vi "auto_detect_arduino.vi"(0 "instr name":string="Arduino Micro" caption="Arduino Board Name", 1 "error in":errorcluster) -> (2 "VISA resource name":refnum<visa-resource-name>, 3 "status":bool, 4 "error out":errorcluster)   [LabVIEW 2013]
uses:
  <vilib>/Instr/_visa.llb/VISA Find Search Mode.ctl
  <vilib>/regexp/Match Regular Expression.xnode
panel:
  # "Auto Detect ARDUINO"
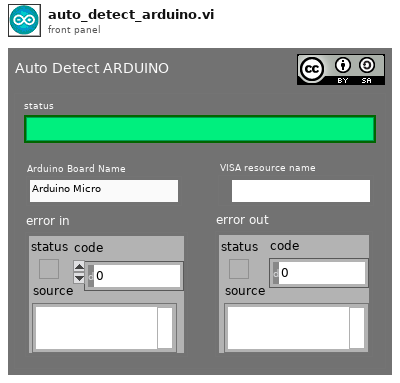
[diagram p1: front panel]
types:
  T1 = typedef "VISA Find Search Mode.ctl" = u32
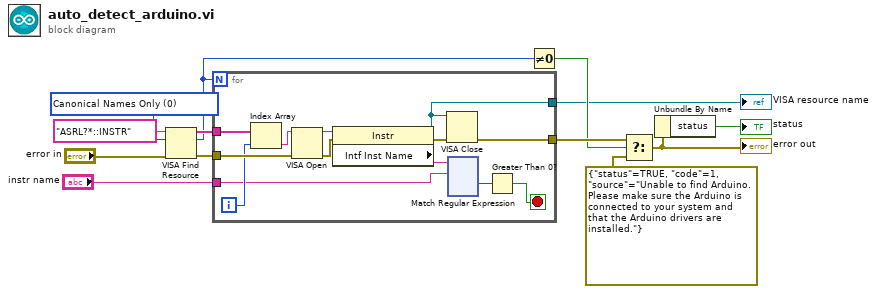
[diagram p0: block diagram]
diagram:
  w1 = T1 0 items=["Canonical Names Only"=0, "Aliases Only"=2, "Include Matching Aliases"=3, "Include All Aliases"=4] ("Search Mode")
  n1 = VISA Find Resource(8:"error in", 10:w1, 11:"ASRL?*::INSTR" ("expression (\"?*\")")) -> (0:w3:errorcluster, 2:w2:u32, 3:w4:string[])
  n2 = for {
    N: w2 -> [_]
    tunnel: w4 -> [w26]
    tunnel: w3 -> [w25]
    tunnel: [w17] -> w7
    tunnel: [w24] -> w13
    tunnel: "instr name" -> [w14]
    i -> [w23]
    stop <- w15 stop-if-true
    n3 = Index Array(array=w26, index=w23) -> (element=w22:string)
    n4 = VISA Open(error in (no error)=w25, VISA resource name=w22) -> (VISA resource name=w21:refnum<visa-resource-name>, error out=w20:errorcluster)  [unwired: 3 in]
    n5 = property class="Instr"(reference=w21, error in=w20) -> (reference out=w17:refnum<visa-resource-name>, error out=w19:errorcluster, "Intf Inst Name"=w16:string)
    n6 = VISA Close(VISA resource name=w17, error in (no error)=w19) -> (error out=w24:errorcluster)
    n7 = xnode "Match Regular Expression"("input string"=w16, "regular expression"=w14) -> ("offset past match"=w18:i32)  [unwired: 4 in, 4 out]
    n8 = Greater Than 0?(x=w18) -> (x > 0?=w15:bool)
  }
  "VISA resource name" <- w7
  n9 = Not Equal To 0?(x=w2) -> (x != 0?=w11:bool)
  n10 = Select(t=w13, s=w11, f=errorcluster {"status"=TRUE, "code"=1, "source"="Unable to find Arduino.  Please make sure the Arduino is connected to your system and that the Arduino drivers are installed."}) -> (s? t:f=w10:errorcluster)
  "error out" <- w10
  n11 = Unbundle By Name(w10) -> ("status"=→"status":bool)
